vi "Request Reply Test.vi"() -> ()   [LabVIEW 2020, in "VectoScratch.lvlib"]
uses:
  VectoScratch.lvlib
  Vecto/TCPMessaging/TCPMessaging.lvclass
  Vecto/proto/TcpClientHello/Data.ctl
  Vecto/proto/TcpClientHello/TcpClientHello.lvlib
  Vecto/SequenceCountService/SequenceCountService.lvclass
  RequestReply Message Handler/RequestReply Message Handler.lvclass
  Vecto/TCPMessageService/TCPMessageAPI.lvclass
  f43fa4b8-9013-4cdb-9f53-d6588b84612f.vi
  19c59f3d-4438-4bbc-9f5b-90826cadd21a.vi
  C:/dev/lv20CE/relink/lv-vecto/Vecto/TCPMessageHandler/TCPMessageHandler.lvclass
panel:
  out "Response":dbl
  in  "B":dbl=6.0
  in  "A":dbl=7.0
  out "Server Error":errorcluster
  out "Client Error":errorcluster
  # "Set A & B and then run the VI to perform multiplication via Request / Reply. The server sends the operands to the client and awaits the response."
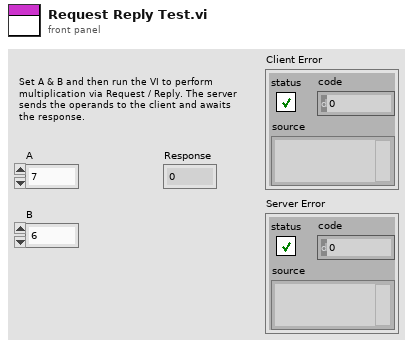
[diagram p1: front panel]
types:
  T1 = typedef "TcpClientHello.lvlib/Data.ctl" = cluster{"node_id":u32, "system":string, "cluster":string, "node_name":string, "app_version":string, "config_version":string}
  T2 = typedef "TcpPayload.lvlib/Data.ctl" = cluster{"target_node":u32, "target_task":u32, "source_id":u32, "sequence":u32, "timestamp":u64, "type":string, "payload":u8[]}
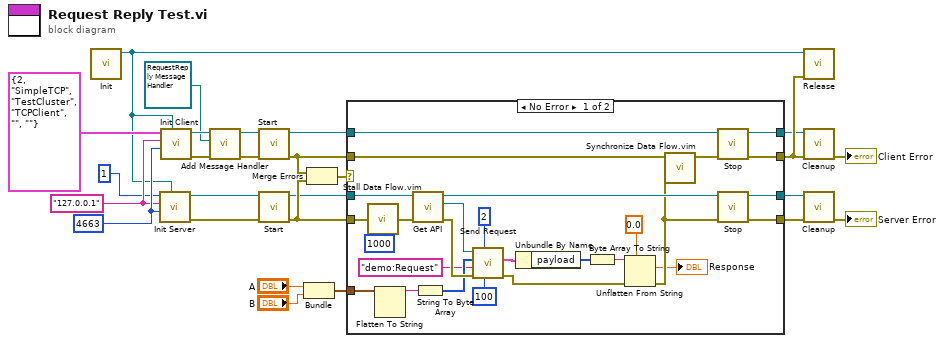
[diagram p0: block diagram]
diagram:
  w25 = u16 4663 ("Bind Port")
  w24 = "127.0.0.1" ("Bind Address")
  n1 = call "Init.vi"() -> ("SequenceCountService out"=w9:refnum<class "SequenceCountService.lvclass">)  [unwired: 10 in, 1 out]
  n2 = call "Init Server.vi"("SequenceCountService"=w9, "Bind Port"=w25, "Bind Address"=w24, "Node ID"=u32 1) -> ("error out"=w1:errorcluster, "TCPMessaging out"=w2:refnum<class "TCPMessaging.lvclass">)  [unwired: 6 in]
  n3 = call "Init Client.vi"("SequenceCountService"=w9, "Remote Port"=w25, "Remote Address"=w24, "Client Info"=T1 {"node_id"=2, "system"="SimpleTCP", "cluster"="TestCluster", "node_name"="TCPClient", "app_version"="", "config_version"=""}) -> ("error out"=w7:errorcluster, "TCPMessaging out"=w8:refnum<class "TCPMessaging.lvclass">)  [unwired: 6 in]
  n4 = call "Add Message Handler.vi"("error in (no error)"=w7, "TCPMessageHandler"=refnum<class "RequestReply Message Handler.lvclass"> refnum ("VectoScratch.lvlib:RequestReply Message Handler.lvclass"), "TCPMessaging in"=w8) -> ("error out"=w21:errorcluster, "TCPMessaging out"=w22:refnum<class "TCPMessaging.lvclass">)  [unwired: 7 in]
  n5 = call "Start.vi"("error in (no error)"=w21, "TCPMessaging in"=w22) -> ("error out"=w19:errorcluster, "TCPMessaging out"=w16:refnum<class "TCPMessaging.lvclass">)  [unwired: 8 in]
  n6 = call "Start.vi"("error in (no error)"=w1, "TCPMessaging in"=w2) -> ("error out"=w18:errorcluster, "TCPMessaging out"=w17:refnum<class "TCPMessaging.lvclass">)  [unwired: 8 in]
  n7 = Bundle("A"="A", "B"="B") -> (w3:cluster{"A":dbl, "B":dbl})  [unwired: 1 in]
  n8 = Merge Errors(w19, w18) -> (w20:errorcluster)
  n9 = case shown="No Error" w20 {
    tunnel: w19 -> [w43 w57]
    tunnel: w18 -> [w51 w56]
    tunnel: w17 -> [w52 w55]
    tunnel: w16 -> [w46 w54]
    tunnel: [w29 w57] -> w26
    tunnel: [w30 w56] -> w13
    tunnel: [w48 w55] -> w14
    tunnel: [w49 w54] -> w15
    tunnel: w3 -> [w47 _]
    frame No Error {
      n10 = call "Stall Data Flow.vim"("value in"=w51, "milliseconds to wait"=u32 1000) -> ("value out"=w32:errorcluster)  [unwired: 1 out]
      n11 = Flatten To String(anything=w47) -> (data string=w40:string)  [unwired: 3 in, 2 out]
      n12 = call "Get API.vi"("error in (no error)"=w32, "TCPMessaging in"=w52) -> ("error out"=w53:errorcluster, "TCP Messaging API"=w45:refnum<class "TCPMessageAPI.lvclass">, "TCPMessaging out"=w50:refnum<class "TCPMessaging.lvclass">)  [unwired: 7 in]
      n13 = String To Byte Array(string=w40) -> (unsigned byte array=w39:u8[])
      n14 = call "Send Request.vi"("Timeout mS (5000)"=100, "Target Node"=u32 2, "error in (no error)"=w53, "Type"="demo:Request", "Payload"=w39, "TCPMessageAPI in"=w45) -> ("error out"=w36:errorcluster, "Reply"=w41:T2)  [unwired: 3 in, 1 out]
      n15 = Unbundle By Name(w41) -> ("payload"=w38:u8[])
      n16 = Byte Array To String(unsigned byte array=w38) -> (string=w37:string)
      n17 = Unflatten From String(type=0.0, binary string=w37, error in (no error)=w36) -> (value=→"Response":dbl, error out=w35:errorcluster)  [unwired: 2 in, 1 out]
      n18 = call "Synchronize Data Flow.vim"("input 4"=w35, "input 1"=w43) -> ("output 1"=w42:errorcluster)  [unwired: 2 in, 3 out]
      n19 = call "Stop.vi"("error in (no error)"=w42, "TCPMessaging in"=w46) -> ("error out"=w29:errorcluster, "TCPMessaging out"=w49:refnum<class "TCPMessaging.lvclass">)  [unwired: 8 in]
      n20 = call "Stop.vi"("error in (no error)"=w35, "TCPMessaging in"=w50) -> ("error out"=w30:errorcluster, "TCPMessaging out"=w48:refnum<class "TCPMessaging.lvclass">)  [unwired: 8 in]
    }
    frame Error {
    }
  }
  n21 = call "Release.vi"("error in (no error)"=w26, "SequenceCountService in"=w9) -> ()  [unwired: 9 in, 1 out]
  n22 = call "Cleanup.vi"("error in (no error)"=w26, "TCPMessaging in"=w15) -> ("error out"=→"Client Error":errorcluster)  [unwired: 9 in]
  n23 = call "Cleanup.vi"("error in (no error)"=w13, "TCPMessaging in"=w14) -> ("error out"=→"Server Error":errorcluster)  [unwired: 9 in]
